vi "login.vi"() -> ()   [LabVIEW 2012]
uses:
  <vilib>/Utility/file.llb/Read From Spreadsheet File (string).vi
panel:
  in  "password":string
  in  "username":T1
  in  "quite":T2
  in  "logion":T3
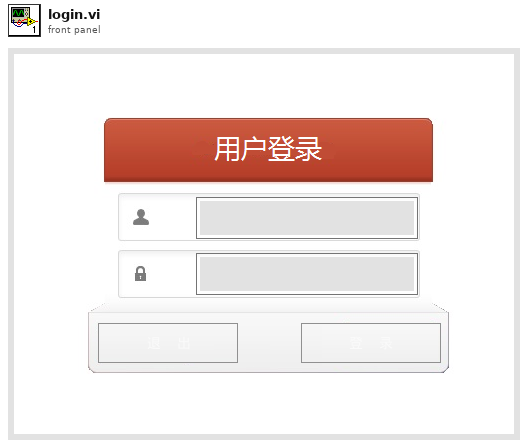
[diagram p1: front panel]
types:
  T1 = typedef "用户输入.ctl" = string
  T2 = typedef "退出.ctl" = bool
  T3 = typedef "登录.ctl" = bool
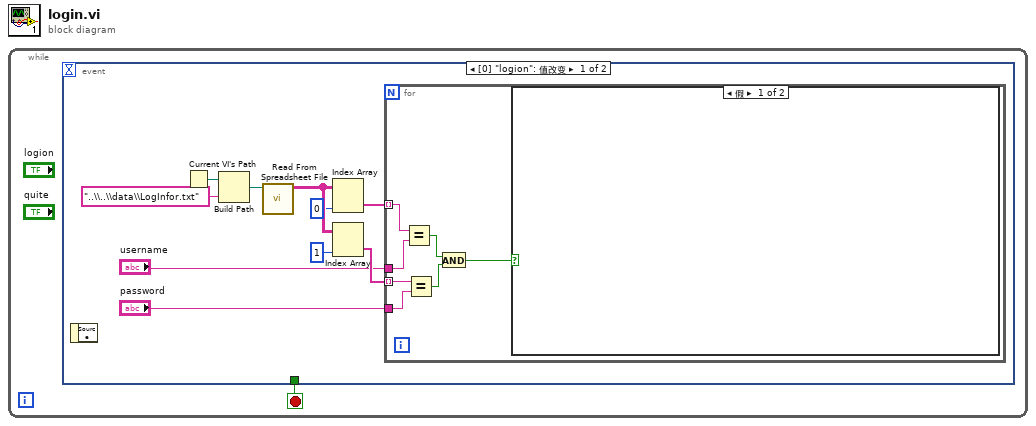
[diagram p0: block diagram]
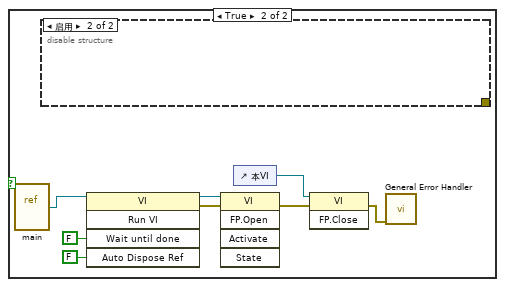
[diagram p2: hidden frame]
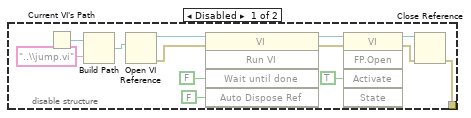
[diagram p3: hidden frame]
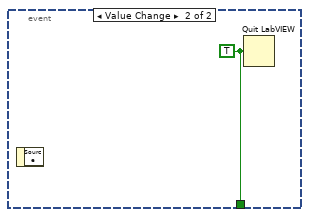
[diagram p4: hidden frame]
diagram:
  n1 = while {
    stop <- w1 stop-if-true
    n2 = event shown="[0] \"logion\": 值改变" {
      selector: _ -> [_ _]
      dyn-events: _ -> [_ _]
      timeout: _ -> [_ _]
      tunnel: [_ w40] -> w1
      event Value Change {
        n3 = event-data() -> ()  [unwired: 1 in, 1 out]
        n4 = Current VI's Path() -> (path=w11:path)
        n5 = Build Path(base path=w11, name or relative path="..\\..\\data\\LogInfor.txt" ("名称或相对路径")) -> (appended path=w9:path)
        n6 = call-poly <vilib>:"Read From Spreadsheet File.vi"("file path (dialog if empty)"=w9) -> ("all rows"=w7:string[][])  [unwired: 6 in, 4 out]
        n7 = Index Array(array=w7, index (col)=0 ("禁用的索引 (列)")) -> (element=w8:string[])  [unwired: 1 in]
        n8 = Index Array(array=w7, index (col)=1 ("禁用的索引 (列)")) -> (element=w6:string[])  [unwired: 1 in]
        n9 = for {
          tunnel: w8 -> [w18] mode=indexing
          tunnel: w6 -> [w17] mode=indexing
          tunnel: "username" -> [w16]
          tunnel: "password" -> [w15]
          n10 = Equal?(x=w18, y=w16) -> (x = y?=w14:bool)
          n11 = Equal?(x=w17, y=w15) -> (x = y?=w13:bool)
          n12 = And(x=w14, y=w13) -> (x .and. y?=w12:bool)
          n13 = case shown="假" w12 {
            frame False {
            }
            frame True {
              n14 = vi-ref "main.vi"() -> (w25:refnum<vi>)
              n15 = disable-structure shown="启用" {
                disable-tunnel: [w27 _] -> _
                frame Disabled {
                  n16 = Current VI's Path() -> (path=w38:path)
                  n17 = Build Path(base path=w38, name or relative path="..\\jump.vi" ("名称或相对路径")) -> (appended path=w37:path)
                  n18 = Open VI Reference(vi path=w37) -> (vi reference=w36:refnum<vi>, error out=w35:errorcluster)  [unwired: 5 in]
                  n19 = invoke class="VI" method="Run VI"(reference=w36, error in=w35, "Wait until done"=FALSE ("结束前等待"), "Auto Dispose Ref"=FALSE ("自动销毁引用")) -> (reference out=w32:refnum<vi>, error out=w31:errorcluster)  [unwired: 1 in, 3 out]
                  n20 = invoke class="VI" method="FP.Open"(reference=w32, error in=w31, "Activate"=TRUE ("激活？")) -> (reference out=w28:refnum<vi>, error out=w29:errorcluster)  [unwired: 2 in, 3 out]
                  n21 = Close Reference(reference=w28, error in (no error)=w29) -> (error out=w27:errorcluster)
                }
                frame Enabled {
                }
              }
              n22 = invoke class="VI" method="Run VI"(reference=w25, "Wait until done"=FALSE ("结束前等待"), "Auto Dispose Ref"=FALSE ("自动销毁引用")) -> (reference out=w22:refnum<vi>, error out=w21:errorcluster)  [unwired: 2 in, 3 out]
              n23 = invoke class="VI" method="FP.Open"(reference=w22, error in=w21) -> (error out=w20:errorcluster)  [unwired: 3 in, 4 out]
              n24 = control-ref of="本VI"() -> (w26:refnum<vi>)
              n25 = invoke class="VI" method="FP.Close"(reference=w26, error in=w20) -> (error out=w19:errorcluster)  [unwired: 1 in, 2 out]
              n26 = call <vilib>:"General Error Handler.vi"("error in (no error)"=w19) -> ()  [unwired: 10 in, 5 out]
            }
          }
        }
      }
      event Value Change {
        w40 = TRUE ("退出？(T)")
        n27 = event-data() -> ()  [unwired: 1 in, 1 out]
        n28 = Quit LabVIEW(quit? (T)=w40) -> ()
      }
    }
  }
